vi "Populate String with INI Variable.vi"(5 "Section":string, 6 "Error in":errorcluster caption="Error in (no error)", 7 "depth":i32, 8 "variable History":string[](array[string]), 9 "String might with variables":string) -> (0 "Error out":errorcluster, 3 "String out":string)   [LabVIEW 2017, in "INI-Static-Variable-Support.lvlib"]
uses:
  INI-Static-Variable-Support.lvlib
  <userlib>/_NEVSTOP/Communicable State Machine(CSM)/Communicable State Machine.lvlib
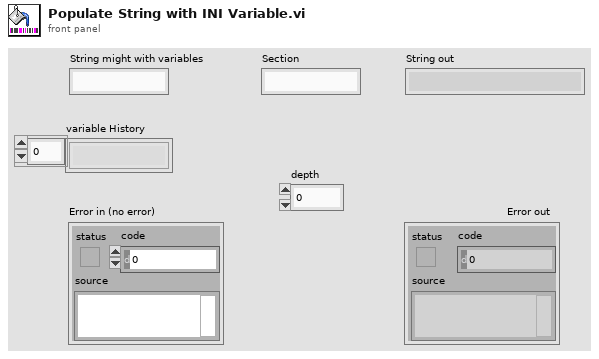
[diagram p1: front panel]
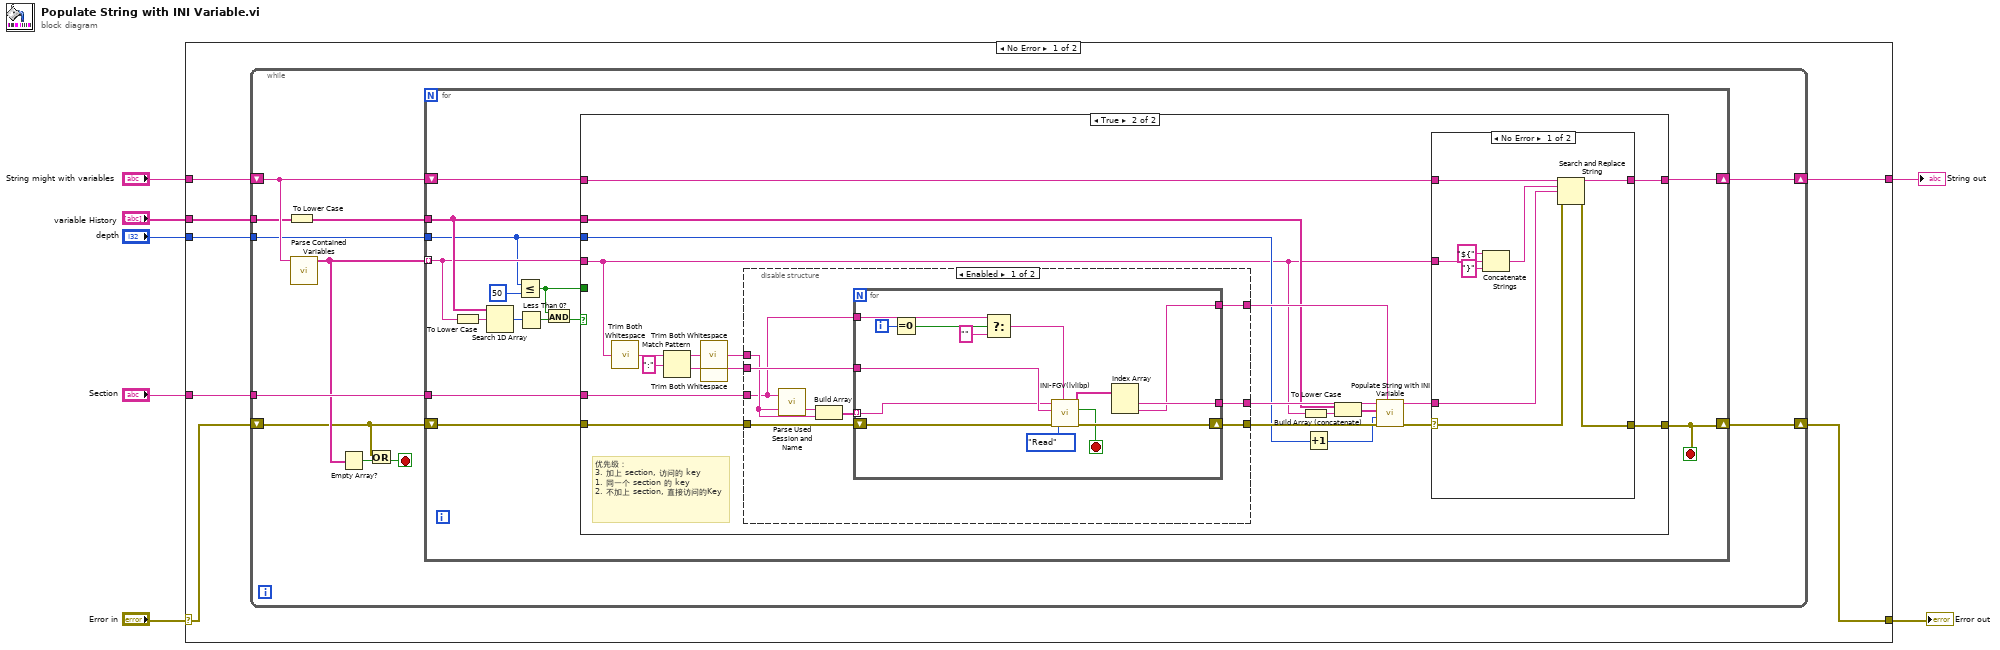
[diagram p0: block diagram]
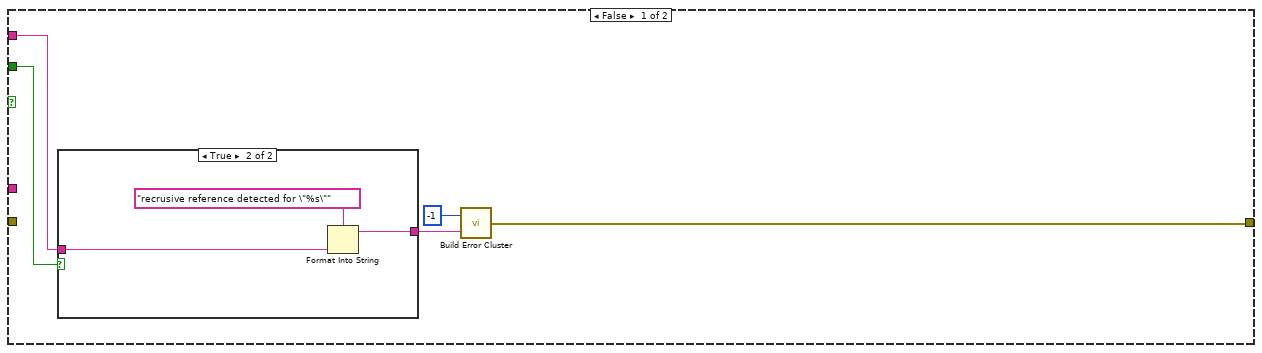
[diagram p2: hidden frame]
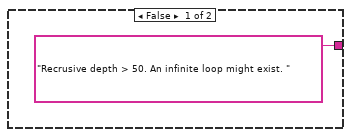
[diagram p3: hidden frame]
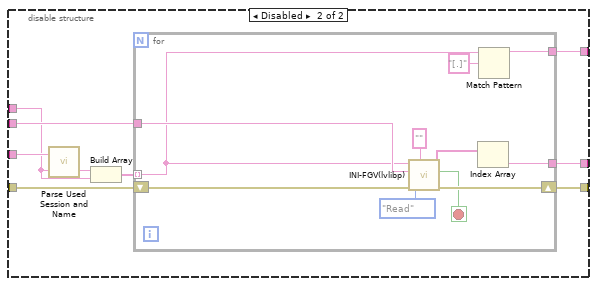
[diagram p4: hidden frame]
diagram:
  n1 = case shown="No Error" "Error in" {
    selector: "Error in" -> [w10 w125]
    tunnel: [w14 w124] -> w7
    tunnel: "Section" -> [w13 _]
    tunnel: "String might with variables" -> [w12 w124]
    tunnel: [w9 w125] -> w3
    tunnel: "variable History" -> [w11 _]
    tunnel: "depth" -> [w8 _]
    frame No Error {
      n2 = while {
        shift-right: [w24] -> w14
        shift-left: w12 -> [w22]
        tunnel: w13 -> [w25]
        tunnel: w11 -> [w19]
        shift-right: [w20] -> w9
        shift-left: w10 -> [w16]
        tunnel: w8 -> [w15]
        stop <- w17 stop-if-true
        n3 = To Lower Case(string=w19) -> (all lower case string=w18:string[])
        n4 = call "Parse Contained Variables.vi"("String"=w22) -> ("Contained Variables"=w21:string[])  [unwired: 10 in]
        n5 = Empty Array?(array=w21) -> (empty?=w23:bool)
        n6 = Or(x=w16, y=w23) -> (x .or. y?=w17:bool)
        n7 = for {
          tunnel: w21 -> [w35] mode=indexing
          shift-right: [w38] -> w24
          shift-left: w22 -> [w39]
          tunnel: w25 -> [w37]
          tunnel: w18 -> [w36]
          shift-right: [w32] -> w20
          shift-left: w16 -> [w31]
          tunnel: w15 -> [w29]
          stop <- w32 stop-if-true
          n8 = To Lower Case(string=w35) -> (all lower case string=w34:string)
          n9 = Search 1D Array(1D array=w36, element=w34) -> (index of element=w33:i32)  [unwired: 1 in]
          n10 = Less Or Equal?(x=w29, y=50) -> (x <= y?=w27:bool)
          n11 = Less Than 0?(x=w33) -> (x < 0?=w26:bool)
          n12 = And(x=w27, y=w26) -> (x .and. y?=w30:bool)
          n13 = case shown="True" w30 {
            tunnel: w39 -> [_ w70]
            tunnel: [_ w69] -> w38
            tunnel: [w44 w68] -> w32
            tunnel: w37 -> [_ w67]
            tunnel: w36 -> [_ w54]
            tunnel: w35 -> [w42 w49]
            tunnel: w31 -> [_ w52]
            tunnel: w29 -> [_ w51]
            tunnel: w27 -> [w40 _]
            frame False {
              n14 = case shown="True" w40 {
                tunnel: w42 -> [_ w47]
                tunnel: ["Recrusive depth > 50. An infinite loop might exist. " w46] -> w41
                frame False {
                }
                frame True {
                  n15 = Format Into String(format string="recrusive reference detected for \"%s\"", w47) -> (resulting string=w46:string)  [unwired: 2 in, 1 out]
                }
              }
              n16 = call <userlib>:"Build Error Cluster.vi"("String to Prepend to Source (\"\")"=w41, "Code"=-1 ("code")) -> ("error out"=w44:errorcluster)
            }
            frame True {
              # "优先级：\n3. 加上 section, 访问的 key \n1. 同一个 section 的 key\n2. 不加上 section, 直接访问的Key"
              n17 = call <userlib>:"Trim Both Whitespace.vi"("String"=w49) -> ("Trimmed String"=w62:string)  [unwired: 1 in]
              n18 = Match Pattern(string=w62, regular expression=":") -> (before substring=w65:string, after substring=w64:string)  [unwired: 1 in, 2 out]
              n19 = call <userlib>:"Trim Both Whitespace.vi"("String"=w65) -> ("Trimmed String"=w56:string)  [unwired: 1 in]
              n20 = call <userlib>:"Trim Both Whitespace.vi"("String"=w64) -> ("Trimmed String"=w63:string)  [unwired: 1 in]
              n21 = disable-structure shown="Enabled" {
                disable-tunnel: w67 -> [w71 w102]
                disable-tunnel: w63 -> [w79 w101]
                disable-tunnel: [w78 w100] -> w61
                disable-tunnel: [w77 w99] -> w60
                disable-tunnel: [w76 w98] -> w58
                disable-tunnel: w56 -> [w73 w95]
                disable-tunnel: w52 -> [w72 w94]
                frame Enabled {
                  n22 = call "Parse Used Session and Name.vi"("name"=w73, "Section Name(\"\" as Default)"=w71) -> ("used name"=w74:string)  [unwired: 1 in]
                  n23 = Build Array(w74, w73) -> (w75:string[])
                  n24 = for {
                    tunnel: w79 -> [w93]
                    tunnel: [w85] -> w78
                    tunnel: [w90] -> w77
                    tunnel: w75 -> [w88] mode=indexing
                    shift-right: [w89] -> w76
                    shift-left: w72 -> [w86]
                    tunnel: w71 -> [w84]
                    i -> [w83]
                    stop <- w87 stop-if-true
                    n25 = Equal To 0?(x=w83) -> (x = 0?=w82:bool)
                    n26 = Select(t=w84, s=w82, f="") -> (s? t:f=w80:string)
                    n27 = call "INI-FGV(lvlibp).vi"("Enum"=enum16{"Read", "Write", "Sync"}."Read", "Prefered Section"=w80, "error IN"=w86, ">> Default Value >>"=w93, ">> Variable Name >>"=w88) -> ("error out"=w89:errorcluster, "Key?"=w87:bool, "Array"=w92:string[])  [unwired: 3 in, 1 out]
                    n28 = Index Array(array=w92) -> (element #1=w90:string, element #2=w85:string)  [unwired: 2 in]
                  }
                }
                frame Disabled {
                  n29 = call "Parse Used Session and Name.vi"("name"=w95, "Section Name(\"\" as Default)"=w102) -> ("used name"=w96:string)  [unwired: 1 in]
                  n30 = Build Array(w96, w95) -> (w97:string[])
                  n31 = for {
                    tunnel: w101 -> [w113]
                    tunnel: [w109] -> w100
                    tunnel: [w108] -> w99
                    tunnel: w97 -> [w106] mode=indexing
                    shift-right: [w107] -> w98
                    shift-left: w94 -> [w104]
                    stop <- w105 stop-if-true
                    n32 = call "INI-FGV(lvlibp).vi"("Enum"=enum16{"Read", "Write", "Sync"}."Read", "Prefered Section"="", "error IN"=w104, ">> Default Value >>"=w113, ">> Variable Name >>"=w106) -> ("error out"=w107:errorcluster, "Key?"=w105:bool, "Array"=w111:string[])  [unwired: 3 in, 1 out]
                    n33 = Index Array(array=w111) -> (element=w108:string)  [unwired: 1 in]
                    n34 = Match Pattern(string=w106, regular expression="[.]") -> (before substring=w109:string)  [unwired: 1 in, 3 out]
                  }
                }
              }
              n35 = To Lower Case(string=w49) -> (all lower case string=w53:string)
              n36 = Increment(x=w51) -> (x+1=w50:i32)
              n37 = Build Array (concatenate)(w54, w53) -> (w55:string[])
              n38 = call "Populate String with INI Variable.vi"("Section"=w61, "Error in"=w58, "depth"=w50, "variable History"=w55, "String might with variables"=w60) -> ("Error out"=w57:errorcluster, "String out"=w59:string)  [unwired: 3 in]
              n39 = case shown="No Error" w57 {
                selector: w57 -> [w116 w123]
                tunnel: w70 -> [w120 _]
                tunnel: [w119 _] -> w69
                tunnel: [w118 w123] -> w68
                tunnel: w59 -> [w117 _]
                tunnel: w49 -> [w114 _]
                frame No Error {
                  n40 = Concatenate Strings("${" ("regular expression"), w114, "}" ("regular expression")) -> (w115:string)
                  n41 = Search and Replace String(input string=w120, search string=w115, replace string=w117, error in=w116) -> (result string=w119:string, error out=w118:errorcluster)  [unwired: 4 in, 2 out]
                }
                frame Error {
                }
              }
            }
          }
        }
      }
    }
    frame Error {
    }
  }
  "String out" <- w7
  "Error out" <- w3
